vi "EXDIR-YAML_Recursive_YAML_Lines_to_Dictionary_ATTEMPT2.vi"(9 "End Index":i32, 10 "Start Index":i32, 11 "ENTIRE Array of YAML Lines":string[](array[string])) -> (1 "items":cluster{"key":variant, "value":variant}[](array[cluster]), 3 "dictionary out":T1)   [LabVIEW 2016]
uses:
  <userlib>/_OpenG.lib/dictionary/dictionary.llb/Dictionary Object RefNum__ogtk.ctl
  <userlib>/_OpenG.lib/dictionary/dictionary.llb/Dictionary Object RefNum - Enum__ogtk.ctl
  <userlib>/_OpenG.lib/dictionary/dictionary.llb/Dictionary Update (by scalar value)__ogtk.vi
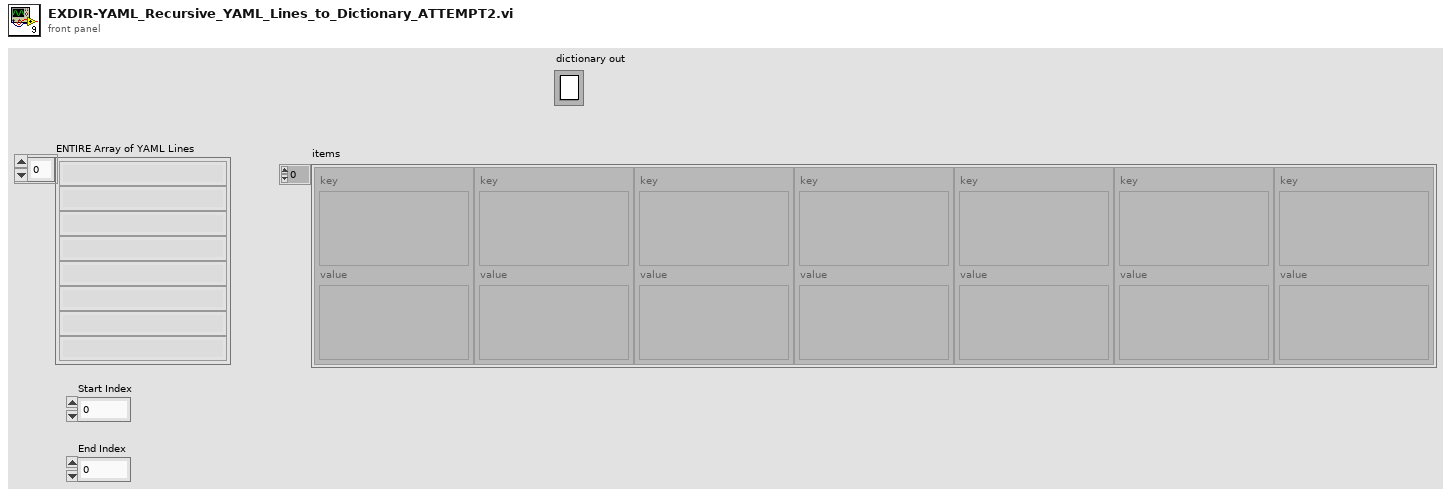
[diagram p1: front panel]
types:
  T1 = typedef "Dictionary Object RefNum__ogtk.ctl" = refnum<k1>
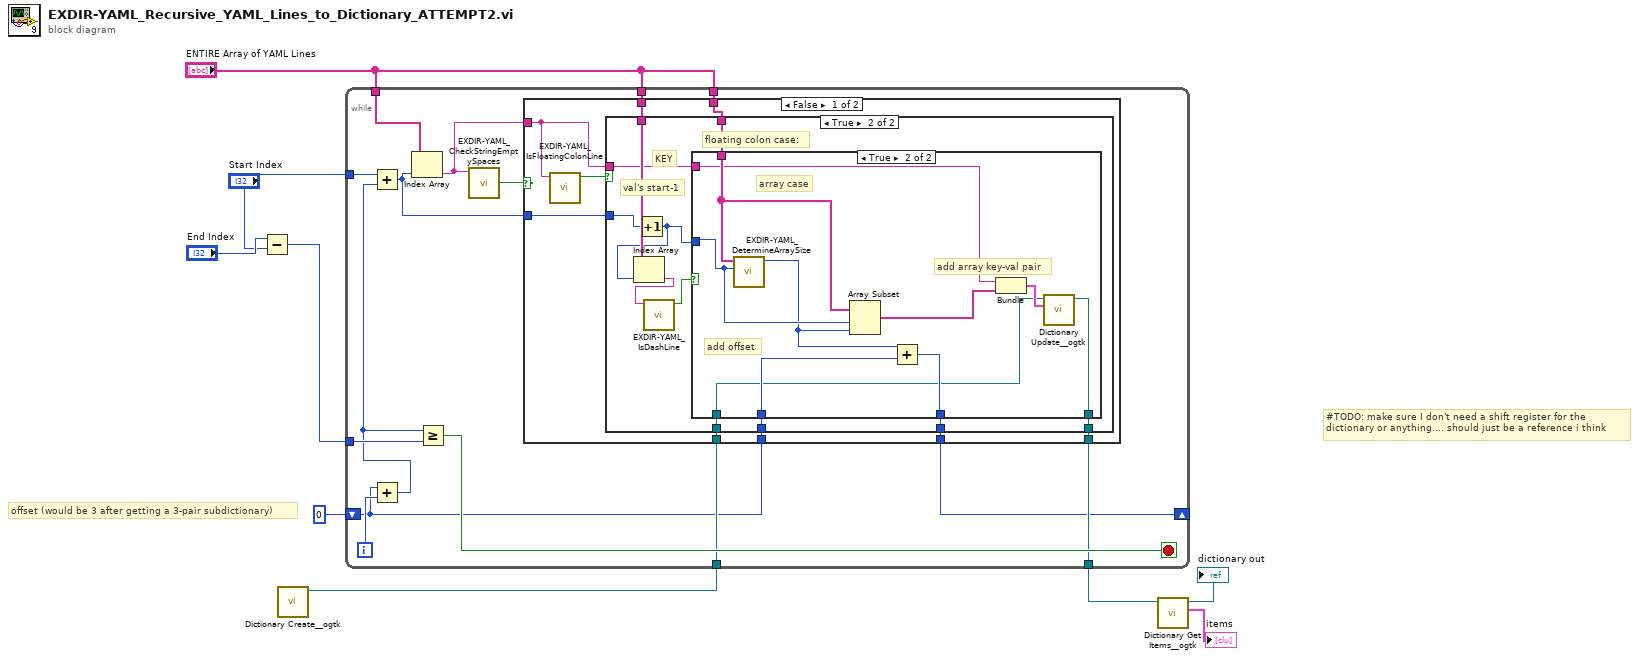
[diagram p0: block diagram]
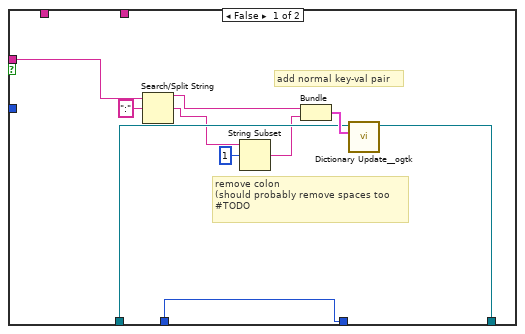
[diagram p2: hidden frame]
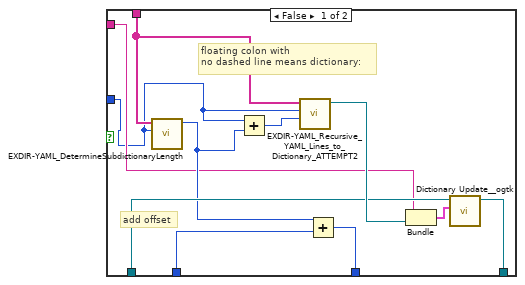
[diagram p3: hidden frame]
diagram:
  # "offset (would be 3 after getting a 3-pair subdictionary)"
  # "#TODO: make sure I don't need a shift register for the\ndictionary or anything.... should just be a reference i think"
  n1 = Subtract(x="End Index", y="Start Index") -> (x-y=w7:i32)
  n2 = call <userlib>:"Dictionary Create__ogtk.vi"() -> ("dictionary out"=w6:T1)  [unwired: 10 in, 1 out]
  n3 = while {
    tunnel: "Start Index" -> [w24]
    tunnel: "ENTIRE Array of YAML Lines" -> [w20]
    tunnel: "ENTIRE Array of YAML Lines" -> [w19]
    tunnel: w7 -> [w18]
    tunnel: w6 -> [w16]
    tunnel: [w15] -> w5
    shift-right: [w11] -> _
    shift-left: 0 -> [w12]
    tunnel: "ENTIRE Array of YAML Lines" -> [w10]
    i -> [w14]
    stop <- w17 stop-if-true
    n4 = Add(x=w12, y=w14) -> (x+y=w13:i32)
    n5 = Add(x=w24, y=w13) -> (x+y=w21:i32)
    n6 = Index Array(array=w19, index=w21) -> (element=w23:string)
    n7 = Greater Or Equal?(x=w13, y=w18) -> (x >= y?=w17:bool)
    n8 = call "EXDIR-YAML_CheckStringEmptySpaces.vi"("String"=w23) -> ("empty or all spaces"=w22:bool)  [unwired: 10 in]
    n9 = case shown="False" w22 {
      tunnel: w23 -> [w32 _]
      tunnel: w21 -> [w31 _]
      tunnel: w20 -> [w30 _]
      tunnel: w16 -> [w29 w77]
      tunnel: [w28 w77] -> w15
      tunnel: w12 -> [w27 w76]
      tunnel: [w26 w76] -> w11
      tunnel: w10 -> [w25 _]
      frame False {
        n10 = call "EXDIR-YAML_IsFloatingColonLine.vi"("Line"=w32) -> ("line ends with floating colon"=w33:bool)  [unwired: 10 in]
        n11 = case shown="True" w33 {
          tunnel: w32 -> [w43 w45]
          tunnel: w31 -> [_ w47]
          tunnel: w30 -> [_ w54]
          tunnel: w29 -> [w39 w53]
          tunnel: [w38 w52] -> w28
          tunnel: w27 -> [w37 w51]
          tunnel: [w37 w50] -> w26
          tunnel: w25 -> [_ w48]
          frame False {
            # "remove colon\n(should probably remove spaces too\n#TODO"
            # "add normal key-val pair"
            n12 = Search/Split String(string=w43, search string/char (-)=":") -> (substring before match=w41:string, match + rest of string=w35:string)  [unwired: 1 in, 1 out]
            n13 = String Subset(string=w35, offset (0)=1) -> (substring=w34:string)  [unwired: 1 in]
            n14 = Bundle(w41, w34) -> (w40:cluster{string, string})  [unwired: 1 in]
            n15 = call-poly <userlib>:"Dictionary Update__ogtk.vi"("key-value"=w40, "dictionary"=w39) -> ("dictionary out"=w38:T1)  [unwired: 7 in, 2 out]
          }
          frame True {
            # "KEY"
            # "floating colon case:"
            # "val's start-1"
            n16 = Increment(x=w47) -> (x+1=w46:i32)
            n17 = Index Array(array=w48, index=w46) -> (element=w44:string)
            n18 = call "EXDIR-YAML_IsDashLine.vi"("Line"=w44) -> ("line starts with dash"=w49:bool)  [unwired: 10 in]
            n19 = case shown="True" w49 {
              tunnel: w46 -> [w55 w67]
              tunnel: w54 -> [w65 w69]
              tunnel: w45 -> [w56 w68]
              tunnel: w53 -> [w61 w71]
              tunnel: [w60 w72] -> w52
              tunnel: w51 -> [w58 w74]
              tunnel: [w57 w75] -> w50
              frame False {
                # "floating colon with\nno dashed line means dictionary:"
                # "add offset"
                n20 = call "EXDIR-YAML_DetermineSubdictionaryLength.vi"("start"=w55, "ENTIRE Array of YAML Lines"=w65) -> ("Length"=w59:i32)  [unwired: 8 in, 1 out]
                n21 = Add(x=w55, y=w59) -> (x+y=w64:i32)
                n22 = call "EXDIR-YAML_Recursive_YAML_Lines_to_Dictionary_ATTEMPT2.vi"("End Index"=w64, "Start Index"=w55, "ENTIRE Array of YAML Lines"=w65) -> ("dictionary out"=w63:T1)  [unwired: 7 in, 1 out]
                n23 = Add(x=w59, y=w58) -> (x+y=w57:i32)
                n24 = Bundle(w56, "dictionary out"=w63) -> (w62:cluster{string, "dictionary out":T1})  [unwired: 1 in]
                n25 = call-poly <userlib>:"Dictionary Update__ogtk.vi"("key-value"=w62, "dictionary"=w61) -> ("dictionary out"=w60:T1)  [unwired: 7 in, 2 out]
              }
              frame True {
                # "array case"
                # "add array key-val pair"
                # "add offset"
                n26 = call "EXDIR-YAML_DetermineArraySize.vi"("start"=w67, "ENTIRE Array of YAML Lines"=w69) -> ("Length"=w66:i32)  [unwired: 8 in, 1 out]
                n27 = Array Subset(array=w69, index=w67, length=w66) -> (w70:string[])
                n28 = Add(x=w66, y=w74) -> (x+y=w75:i32)
                n29 = Bundle(w68, w70) -> (w73:cluster{string, string[]})  [unwired: 1 in]
                n30 = call-poly <userlib>:"Dictionary Update__ogtk.vi"("key-value"=w73, "dictionary"=w71) -> ("dictionary out"=w72:T1)  [unwired: 7 in, 2 out]
              }
            }
          }
        }
      }
      frame True {
        # "this line is empty, move along"
      }
    }
  }
  n31 = call <userlib>:"Dictionary Get Items__ogtk.vi"("dictionary"=w5) -> ("items"=→"items":cluster{"key":variant, "value":variant}[], "dictionary out"=→"dictionary out":T1)  [unwired: 8 in, 1 out]
